vi "Formatted Delayed Coordinates and Date Time Continued.vi"() -> ()   [LabVIEW 2012]
panel:
  out "String":string="Run To Select A File"
  out "Array":cluster{"Scanned X":dbl, "Scanned Y":dbl}[](array[cluster])
  out "Scanned Y":dbl
  out "Scanned X":dbl
  out "Extract 9":string
  out "Extract 8":string
  out "Extract 8":string
  out "Extract 7":string
  out "Extract 6":string
  out "Extract 5":string
  out "Extract 4":string
  out "Extract 3":string
  out "Extract 2":string
  out "Extract 1":string
  out "Last Read Text":string
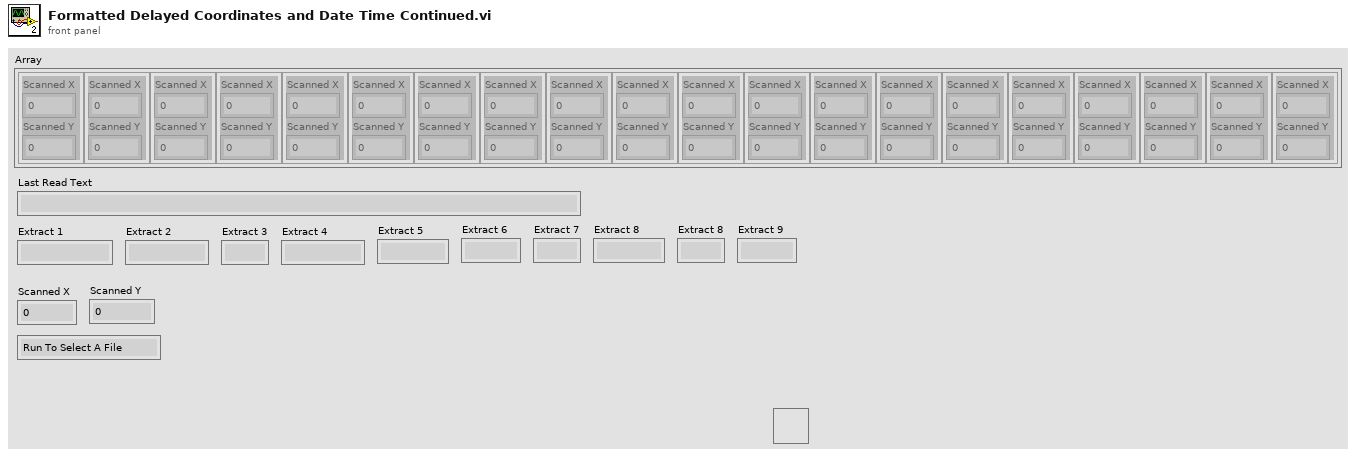
[diagram p1: front panel]
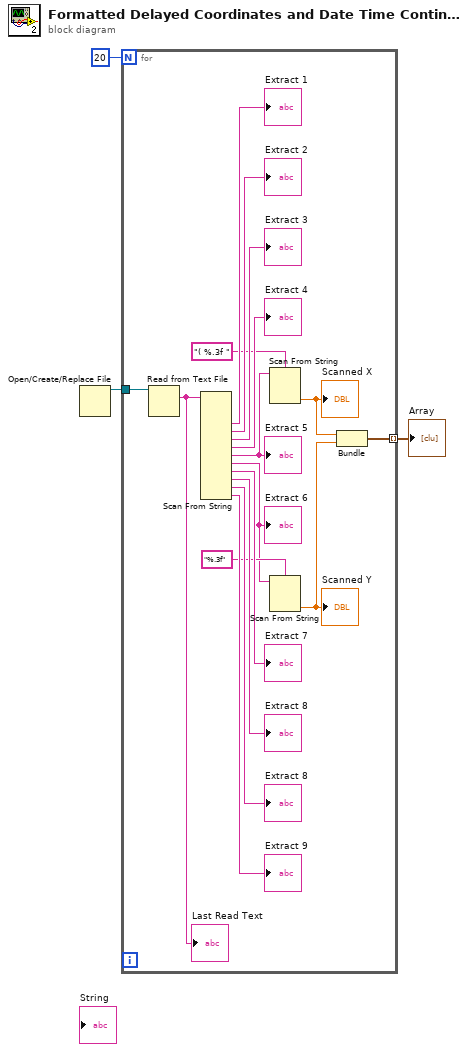
[diagram p0: block diagram]
diagram:
  n1 = Open/Create/Replace File() -> (refnum out=w3:refnum<file>)  [unwired: 6 in, 2 out]
  n2 = for {
    N: 20 -> [_]
    tunnel: w3 -> [w7]
    tunnel: [w4] -> w1 mode=indexing
    n3 = Read from Text File(file (use dialog)=w7) -> (text=w20:string)  [unwired: 3 in, 3 out]
    "Last Read Text" <- w20
    n4 = Scan From String(input string=w20) -> (output 1=→"Extract 1":string, output 2=→"Extract 2":string, output 3=→"Extract 3":string, output 4=→"Extract 4":string, output 5=w8:string, output 6=w9:string, output 7=→"Extract 7":string, output 8=→"Extract 8":string, output 9=→"Extract 8":string, output 10=→"Extract 9":string)  [unwired: 13 in, 3 out]
    "Extract 5" <- w8
    "Extract 6" <- w9
    n5 = Scan From String(format string="( %.3f ", input string=w8) -> (output 1=w6:dbl)  [unwired: 3 in, 3 out]
    "Scanned X" <- w6
    n6 = Scan From String(format string="%.3f", input string=w9) -> (output 1=w5:dbl)  [unwired: 3 in, 3 out]
    "Scanned Y" <- w5
    n7 = Bundle("Scanned X"=w6, "Scanned Y"=w5) -> (w4:cluster{"Scanned X":dbl, "Scanned Y":dbl})  [unwired: 1 in]
  }
  "Array" <- w1
